vi "Post-Build Custom Action.vi"(10 "Variant":variant) -> (0 "error out":errorcluster)   [LabVIEW 2017]
uses:
  <vilib>/Utility/config.llb/Write Key (String).vi
  <vilib>/Utility/config.llb/NI_LVConfig.lvlib
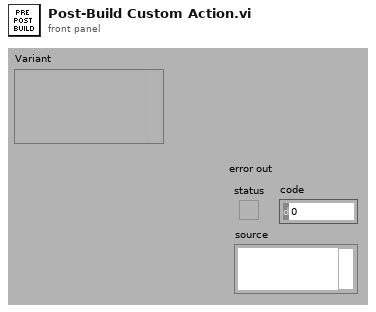
[diagram p1: front panel]
types:
  T1 = typedef "NI_LVConfig.lvlib/Config Data RefNum.ctl" = refnum<k1>
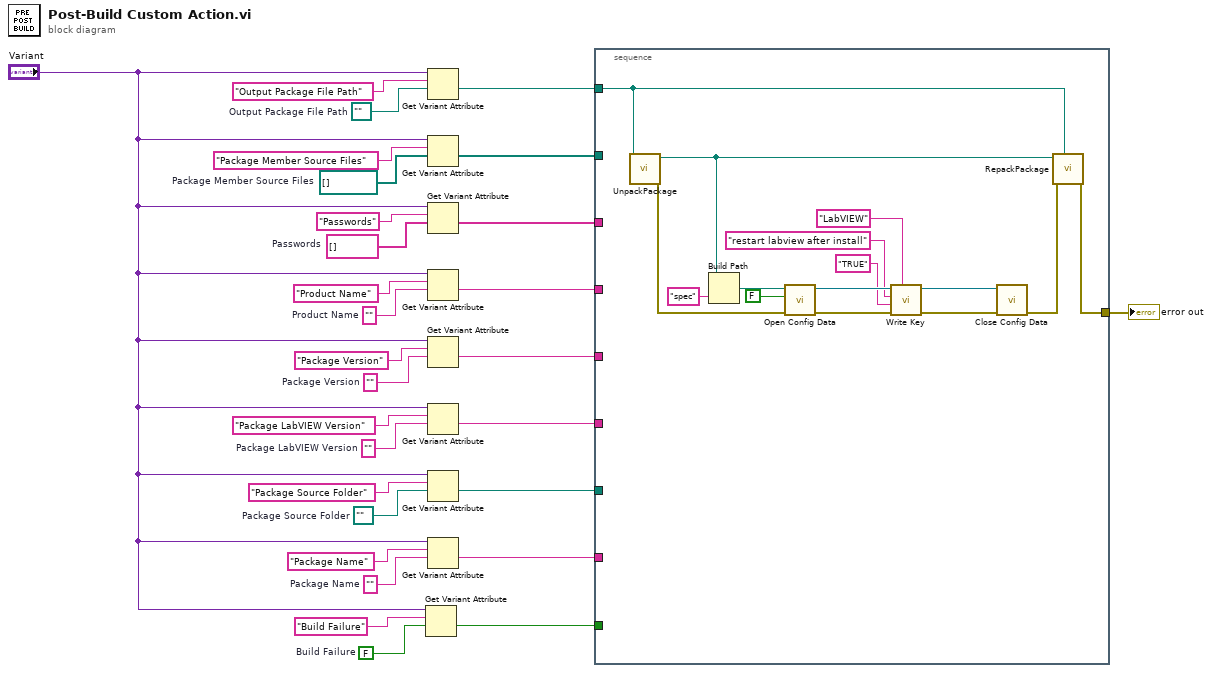
[diagram p0: block diagram]
diagram:
  w4 = FALSE  # Build Failure
  w14 = path ""  # Package Source Folder
  w15 = ""  # Package Name
  w18 = ""  # Package LabVIEW Version
  w20 = ""  # Package Version
  w22 = ""  # Product Name
  w24 = string[] []  # Passwords
  w26 = path[] []  # Package Member Source Files
  w28 = path ""  # Output Package File Path
  n1 = Get Variant Attribute(Variant="Variant", name="Build Failure", default value (empty Variant)=w4) -> (value=w2:bool)  [unwired: 1 in, 3 out]
  n2 = Get Variant Attribute(Variant="Variant", name="Output Package File Path", default value (empty Variant)=w28) -> (value=w13:path)  [unwired: 1 in, 3 out]
  n3 = Get Variant Attribute(Variant="Variant", name="Package Member Source Files", default value (empty Variant)=w26) -> (value=w12:path[])  [unwired: 1 in, 3 out]
  n4 = Get Variant Attribute(Variant="Variant", name="Passwords", default value (empty Variant)=w24) -> (value=w11:string[])  [unwired: 1 in, 3 out]
  n5 = Get Variant Attribute(Variant="Variant", name="Product Name", default value (empty Variant)=w22) -> (value=w10:string)  [unwired: 1 in, 3 out]
  n6 = Get Variant Attribute(Variant="Variant", name="Package Version", default value (empty Variant)=w20) -> (value=w9:string)  [unwired: 1 in, 3 out]
  n7 = Get Variant Attribute(Variant="Variant", name="Package LabVIEW Version", default value (empty Variant)=w18) -> (value=w8:string)  [unwired: 1 in, 3 out]
  n8 = Get Variant Attribute(Variant="Variant", name="Package Source Folder", default value (empty Variant)=w14) -> (value=w7:path)  [unwired: 1 in, 3 out]
  n9 = Get Variant Attribute(Variant="Variant", name="Package Name", default value (empty Variant)=w15) -> (value=w6:string)  [unwired: 1 in, 3 out]
  n10 = stacked-sequence {
    tunnel: w13 -> [w44]
    tunnel: w12 -> [_]
    tunnel: w11 -> [_]
    tunnel: w10 -> [_]
    tunnel: w9 -> [_]
    tunnel: w8 -> [_]
    tunnel: w7 -> [_]
    tunnel: w6 -> [_]
    tunnel: w2 -> [_]
    tunnel: [w30] -> w1
    frame #0 {
      n11 = call "UnpackPackage.vi"("Package File"=w44) -> ("error out"=w32:errorcluster, "Unpacked Package Directory"=w43:path)  [unwired: 8 in, 1 out]
      n12 = Build Path(base path=w43, name or relative path="spec") -> (appended path=w41:path)
      n13 = call <vilib>:"Open Config Data.vi"("error in (no error)"=w32, "create file if necessary (T)"=FALSE, "configuration file path"=w41) -> ("error out"=w39:errorcluster, "refnum"=w38:T1)  [unwired: 6 in, 1 out]
      n14 = call-poly <vilib>:"Write Key.vi"("section"="LabVIEW", "error in (no error)"=w39, "value"="TRUE" ("section"), "key"="restart labview after install", "refnum"=w38) -> ("error out"=w34:errorcluster, "refnum out"=w33:T1)  [unwired: 4 in, 1 out]
      n15 = call <vilib>:"Close Config Data.vi"("error in (no error)"=w34, "refnum"=w33) -> ("error out"=w31:errorcluster)  [unwired: 8 in, 1 out]
      n16 = call "RepackPackage.vi"("Package File (\"\": use name of directory to repack)"=w44, "error in (no error)"=w31, "Directory to repack"=w43) -> ("error out"=w30:errorcluster)  [unwired: 8 in]
    }
  }
  "error out" <- w1
